vi "Acquiring a Signal.vi"() -> ()   [LabVIEW 2011]
doc: "Use this template to generate a signal and display the generated data in a graph. You can use this template with the exercises in the Getting Started with LabVIEW manual.\nNote: LabVIEW enables automatic error handling by default for VIs you create from this template."
uses:
  Instance           1 35Saved   TutorialGenerateDisplay.vit .vi
  <vilib>/express/express shared/transition.llb/Dynamic To Waveform Array.vi
  <vilib>/express/express shared/transition.llb/Waveform Array To Dynamic.vi
  <vilib>/express/express arith-compare/Formula/Block/exnFormulaBlock how many pts in the wave.vi
  <vilib>/express/express shared/ex_Modify Signal Name.vi
  <vilib>/express/express arith-compare/Formula/XNode/ExpressFormulaBlockNode.xnode
panel:
  in  "Knob":dbl(knob) scale=0.0..10.0
  out "Waveform Graph":dynamicdata(graph)
  in  "stop":bool
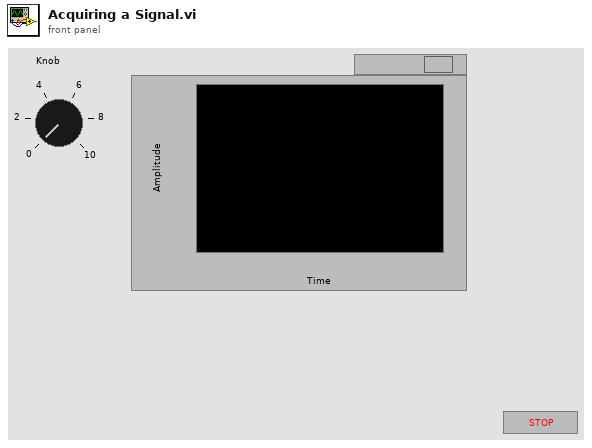
[diagram p1: front panel]
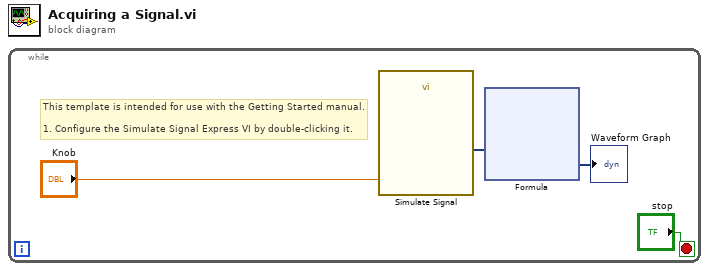
[diagram p0: block diagram]
diagram:
  n1 = while {
    stop <- "stop" stop-if-true
    # "This template is intended for use with the Getting Started manual.\n\n1. Configure the Simulate Signal Express VI by double-clicking it."
    n2 = call "Simulate Signal"("Amplitude"="Knob") -> ("Sawtooth"=w2:dynamicdata)  [unwired: 13 in, 1 out]
    n3 = xnode "Formula"("Sawtooth"=w2) -> ("Result"=→"Waveform Graph":dynamicdata)  [unwired: 1 in, 1 out]
  }
